vi "PRL Queue Reader.vi"(8 "error in (no error)":errorcluster, 11 "timeout in ms (5)":i32=5) -> (0 "error out":errorcluster, 2 "Data":T1, 3 "Has Data?":bool)   [LabVIEW 2018, in "S3DK.lvlib" / "PMU Recorder Light.lvlib"]
uses:
  .S3DK - Copy/PMU Recorder Light/PMU Recorder Light.lvlib
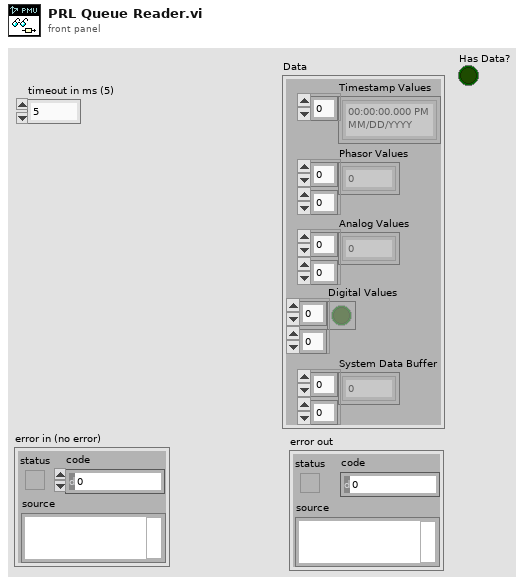
[diagram p1: front panel]
types:
  T1 = cluster{"Timestamp Values":timestamp[], "Phasor Values":csg[][], "Analog Values":sgl[][], "Digital Values":bool[][], "System Data Buffer":sgl[][]}
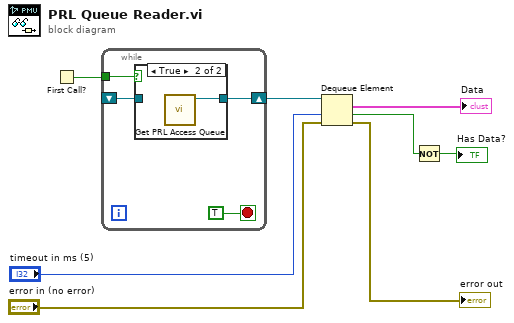
[diagram p0: block diagram]
diagram:
  n1 = First Call?() -> (First Call?: T/F=w8:bool)
  n2 = while {
    tunnel: w8 -> [w11]
    shift-right: [w10] -> w7
    shift-left: _ -> [w9]
    stop <- TRUE stop-if-true
    n3 = case shown="True" w11 {
      tunnel: [w13 w14] -> w10
      tunnel: w9 -> [w13 _]
      frame False {
      }
      frame True {
        n4 = call "Get PRL Access Queue.vi"() -> ("PRL Access Queue"=w14:refnum<queue>)  [unwired: 11 in]
      }
    }
  }
  n5 = Dequeue Element(queue=w7, timeout in ms (-1)="timeout in ms (5)", error in (no error)="error in (no error)") -> (element=→"Data":T1, timed out?=w2:bool, error out=→"error out":errorcluster)  [unwired: 1 out]
  n6 = Not(x=w2) -> (.not. x?=→"Has Data?":bool)
